vi "LJUD U3RAW ConfigU3.vi"(7 "Comm Settings":T3={"Open LabJack "=TRUE, "Address"="1", "FirstFound"=TRUE}, 8 "error in (no error)":errorcluster, 10 "WriteMask0":u8, 11 "Handle In":i32) -> (0 "error out":errorcluster, 3 "Handle Out":i32)   [LabVIEW 2021]
panel:
  in  "DAC Defaults [2]":T1
  in  "Digital Defaults Write [1]":T2
  in  "Local ID [3]":u8
  out "Read Array":u8[](array[numeric]) format="%.0x"
  # "FIOAnalog"
  # "EIOAnalog"
  # "If open is false,\nthen a valid\nhandle must be\npassed in."
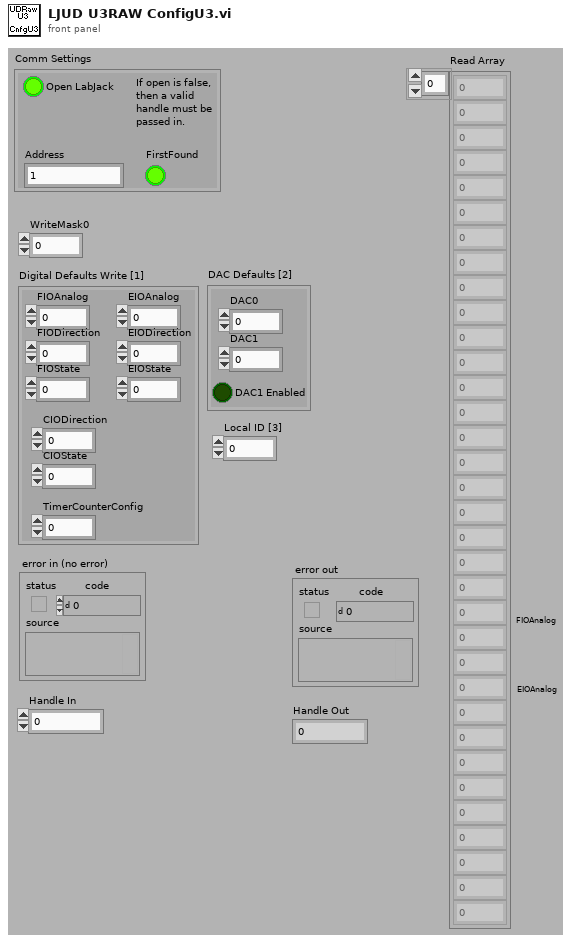
[diagram p1: front panel]
types:
  T1 = cluster{"DAC0":u8, "DAC1":u8, "DAC1 Enabled":bool}
  T2 = cluster{"FIOAnalog":u8, "FIODirection":u8, "FIOState":u8, "EIOAnalog":u8, "EIODirection":u8, "EIOState":u8, "CIODirection":u8, "CIOState":u8, "TimerCounterConfig":u8}
  T3 = cluster{"Open LabJack ":bool, "Address":string, "FirstFound":bool}
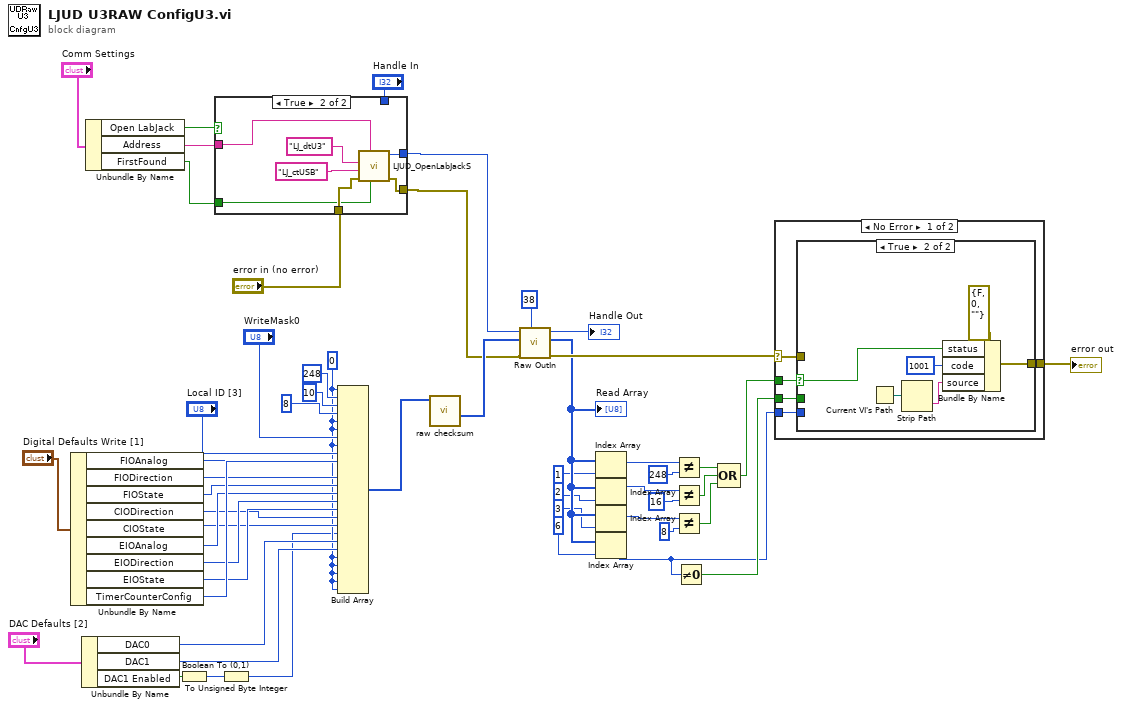
[diagram p0: block diagram]
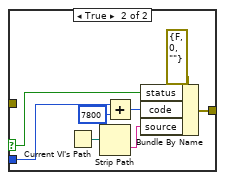
[diagram p3: hidden frame]
diagram:
  w13 = u8 0 ("Input Element")
  n1 = Unbundle By Name("Digital Defaults Write [1]") -> ("FIOAnalog"=w24:u8, "FIODirection"=w23:u8, "FIOState"=w22:u8, "CIODirection"=w18:u8, "CIOState"=w17:u8, "EIOAnalog"=w21:u8, "EIODirection"=w20:u8, "EIOState"=w19:u8, "TimerCounterConfig"=w25:u8)
  n2 = Unbundle By Name("DAC Defaults [2]") -> ("DAC0"=w15:u8, "DAC1"=w14:u8, "DAC1 Enabled"=w12:bool)
  n3 = Unbundle By Name("Comm Settings") -> ("Open LabJack"=w40:bool, "Address"=w39:string, "FirstFound"=w38:bool)
  n4 = Boolean To (0,1)(Boolean=w12) -> (0, 1=w11:i16)
  n5 = case shown="True" w40 {
    tunnel: w39 -> [_ w59]
    tunnel: "error in (no error)" -> [w55 w60]
    tunnel: [w55 w61] -> w43
    tunnel: [w54 w62] -> w42
    tunnel: w38 -> [_ w58]
    tunnel: "Handle In" -> [w54 _]
    frame False {
    }
    frame True {
      n6 = call "LJUD_OpenLabJackS.vi"("FirstFound"=w58, "Address"=w59, "error in"=w60, "ConnectionType"="LJ_ctUSB", "DeviceType"="LJ_dtU3") -> ("error out"=w61:errorcluster, "Handle"=w62:i32)  [unwired: 4 in, 1 out]
    }
  }
  n7 = To Unsigned Byte Integer(number=w11) -> (unsigned 8bit integer=w10:u8)
  n8 = Build Array(w13, u8 248 ("Input Element"), u8 10 ("Input Element"), u8 8 ("Input Element"), w13, w13, "WriteMask0", w13, "Local ID [3]", w25, w24, w23, w22, w21, w20, w19, w18, w17, w10, w15, w14, w13, w13, w13, w13, w13) -> (w50:u8[])
  n9 = call "raw checksum.vi"("Array"=w50) -> ("Array Output"=w48:u8[])  [unwired: 3 in, 7 out]
  n10 = call "Raw OutIn.vi"("# of bytes to read in"=38 ("# of bytes to read"), "error in"=w43, "Raw Out"=w48, "Handle In"=w42) -> ("error out"=w31:errorcluster, "Raw In"=w9:u8[], "Handle Out"=→"Handle Out":i32)  [unwired: 4 in, 1 out]
  "Read Array" <- w9
  n11 = Index Array(array=w9, index=1 ("Index")) -> (element=w4:u8)
  n12 = Index Array(array=w9, index=2 ("Index")) -> (element=w3:u8)
  n13 = Index Array(array=w9, index=3 ("Index")) -> (element=w2:u8)
  n14 = Index Array(array=w9, index=6 ("Index")) -> (element=w1:u8)
  n15 = Not Equal?(x=w4, y=u8 248 ("Input Element")) -> (x != y?=w34:bool)
  n16 = Not Equal?(x=w3, y=u8 16 ("Input Element")) -> (x != y?=w33:bool)
  n17 = Not Equal?(x=w2, y=u8 8 ("Input Element")) -> (x != y?=w32:bool)
  n18 = Not Equal To 0?(x=w1) -> (x != 0?=w29:bool)
  n19 = Compound Arithmetic op=OR(w34, w33, w32) -> (w30:bool)
  n20 = case shown="No Error" w31 {
    selector: w31 -> [w63 w87]
    tunnel: w30 -> [w67 _]
    tunnel: w29 -> [w66 _]
    tunnel: w1 -> [w65 _]
    tunnel: [w64 w87] -> w28
    frame No Error {
      n21 = case shown="True" w67 {
        selector: w67 -> [_ w81]
        tunnel: w66 -> [w71 _]
        tunnel: w65 -> [w70 _]
        tunnel: [w69 w83] -> w64
        tunnel: w63 -> [w68 _]
        frame False {
          n22 = case shown="False" w71 {
            selector: w71 -> [_ w74]
            tunnel: w70 -> [_ w75]
            tunnel: [w72 w73] -> w69
            tunnel: w68 -> [w72 _]
            frame False {
            }
            frame True {
              n23 = Current VI's Path() -> (path=w78:path)
              n24 = Strip Path(path=w78) -> (name=w77:string)  [unwired: 1 out]
              n25 = Add(x=w75, y=7800) -> (x+y=w79:i32)
              n26 = Bundle By Name(cluster=errorcluster {"status"=FALSE, "code"=0, "source"=""} ("error IO"), "status"=w74, "code"=w79, "source"=w77) -> (w73:errorcluster)
            }
          }
        }
        frame True {
          n27 = Current VI's Path() -> (path=w86:path)
          n28 = Strip Path(path=w86) -> (name=w85:string)  [unwired: 1 out]
          n29 = Bundle By Name(cluster=errorcluster {"status"=FALSE, "code"=0, "source"=""} ("error IO"), "status"=w81, "code"=1001, "source"=w85) -> (w83:errorcluster)
        }
      }
    }
    frame Error {
    }
  }
  "error out" <- w28
